vi "Calculator Brainstorming V3.vi"() -> ()   [LabVIEW 2017]
panel:
  in  ".":bool
  in  "÷":bool
  in  "x":bool
  in  "-":bool
  in  "+":bool
  in  "9":bool
  in  "8":bool
  in  "7":bool
  in  "0":bool
  in  "6":bool
  in  "CLEAR":bool
  in  "?":bool
  in  "1":bool
  in  "5":bool
  in  "4":bool
  in  "3":bool
  in  "2":bool
  out "Display":dbl
  # "Don't work:"
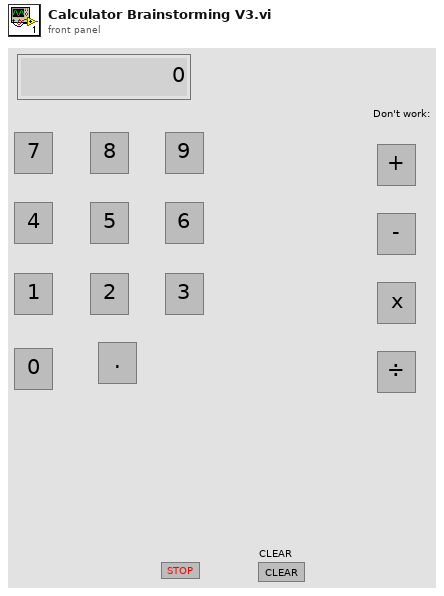
[diagram p1: front panel]
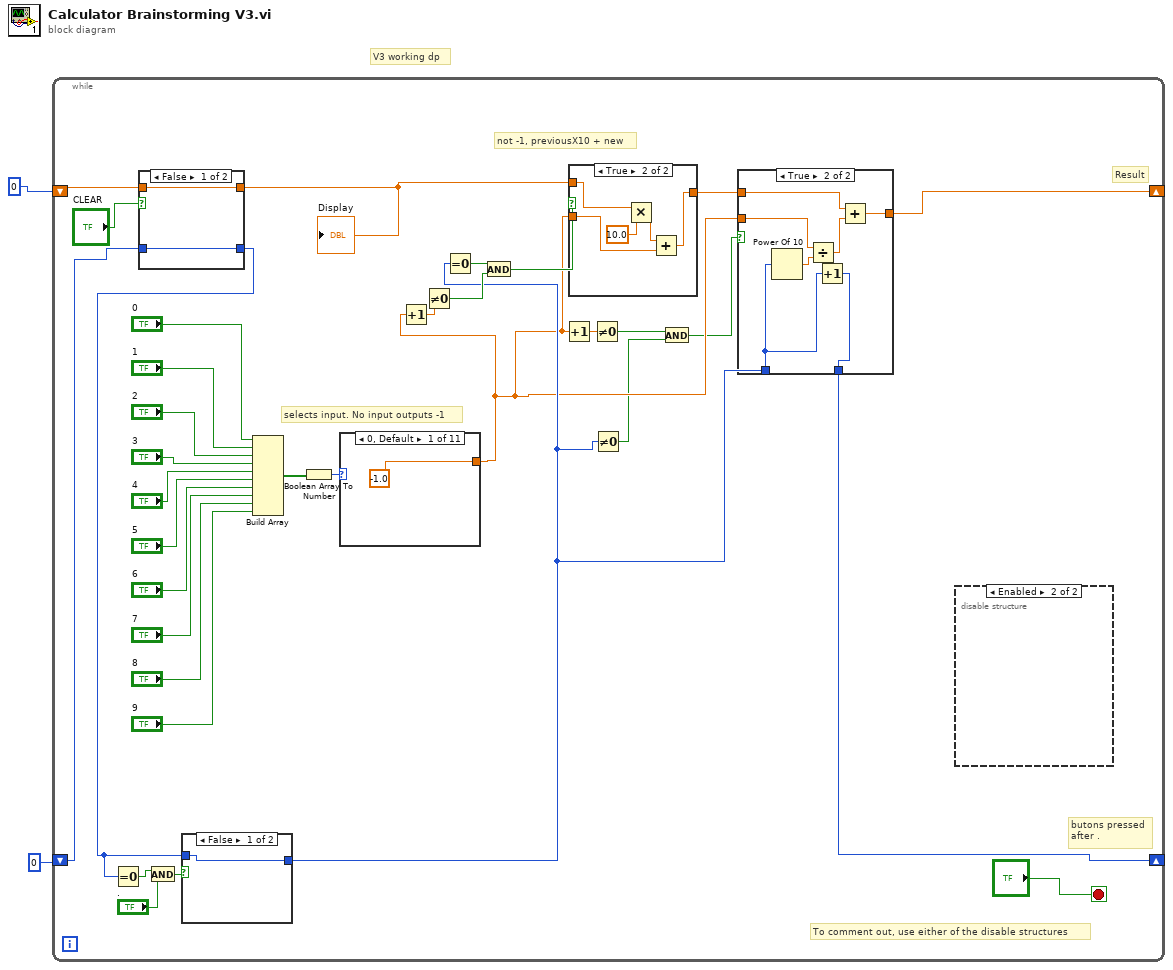
[diagram p0: block diagram]
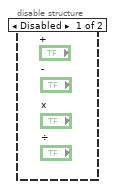
[diagram p2: hidden frame]
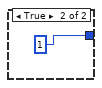
[diagram p5: hidden frame]
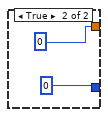
[diagram p6: hidden frame]
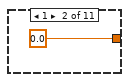
[diagram p7: hidden frame]
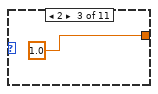
[diagram p8: hidden frame]
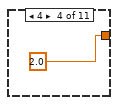
[diagram p9: hidden frame]
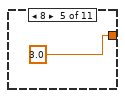
[diagram p10: hidden frame]
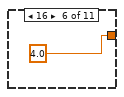
[diagram p11: hidden frame]
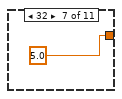
[diagram p12: hidden frame]
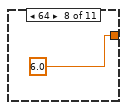
[diagram p13: hidden frame]
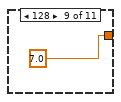
[diagram p14: hidden frame]
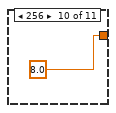
[diagram p15: hidden frame]
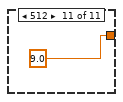
[diagram p16: hidden frame]
diagram:
  # "V3 working dp"
  n1 = while {
    shift-right: [w14] -> _
    shift-left: u8 0 -> [w34]
    shift-right: [w13] -> _
    shift-left: u8 0 -> [w17]
    stop <- "?" stop-if-true
    # "butons pressed\nafter ."
    # "To comment out, use either of the disable structures"
    # "not -1, previousX10 + new"
    # "selects input. No input outputs -1"
    # "Result"
    n2 = case shown="False" "CLEAR" {
      tunnel: [w55 0] -> w16
      tunnel: w34 -> [w55 _]
      tunnel: [w54 0] -> w18
      tunnel: w17 -> [w54 _]
      frame False {
      }
      frame True {
      }
    }
    "Display" <- w16
    n3 = Equal To 0?(x=w18) -> (x = 0?=w20:bool)
    n4 = And(x=w20, y=".") -> (x .and. y?=w21:bool)
    n5 = case shown="False" w21 {
      tunnel: w18 -> [w52 _]
      tunnel: [w52 1] -> w8
      frame False {
      }
      frame True {
      }
    }
    n6 = Build Array("0", "1", "2", "3", "4", "5", "6", "7", "8", "9") -> (w32:bool[])
    n7 = Boolean Array To Number(Boolean array=w32) -> (number=w36:u32)
    n8 = case shown="0, Default" w36 {
      tunnel: [-1.0 0.0 1.0 2.0 3.0 4.0 5.0 6.0 7.0 8.0 9.0] -> w7
      frame 0, Default {
      }
      frame 1 {
      }
      frame 2 {
      }
      frame 4 {
      }
      frame 8 {
      }
      frame 16 {
      }
      frame 32 {
      }
      frame 64 {
      }
      frame 128 {
      }
      frame 256 {
      }
      frame 512 {
      }
    }
    n9 = Increment(x=w7) -> (x+1=w11:dbl)
    n10 = Not Equal To 0?(x=w11) -> (x != 0?=w12:bool)
    n11 = Equal To 0?(x=w8) -> (x = 0?=w10:bool)
    n12 = And(x=w10, y=w12) -> (x .and. y?=w9:bool)
    n13 = Increment(x=w7) -> (x+1=w3:dbl)
    n14 = case shown="True" w9 {
      tunnel: w16 -> [w37 w40]
      tunnel: [w37 w39] -> w15
      tunnel: w7 -> [_ w38]
      frame False {
      }
      frame True {
        n15 = Multiply(x=w40, y=10.0) -> (x*y=w42:dbl)
        n16 = Add(x=w42, y=w38) -> (x+y=w39:dbl)
      }
    }
    n17 = Not Equal To 0?(x=w3) -> (x != 0?=w6:bool)
    n18 = Not Equal To 0?(x=w8) -> (x != 0?=w5:bool)
    n19 = And(x=w6, y=w5) -> (x .and. y?=w4:bool)
    n20 = case shown="True" w4 {
      tunnel: w15 -> [w44 w49]
      tunnel: [w44 w48] -> w14
      tunnel: w8 -> [w43 w46]
      tunnel: w7 -> [_ w47]
      tunnel: [w43 w45] -> w13
      frame False {
      }
      frame True {
        n21 = Power Of 10(x=w46) -> (10^x=w51:dbl)
        n22 = Divide(x=w47, y=w51) -> (x/y=w50:dbl)
        n23 = Increment(x=w46) -> (x+1=w45:i32)
        n24 = Add(x=w49, y=w50) -> (x+y=w48:dbl)
      }
    }
    n25 = disable-structure shown="Enabled" {
      frame Disabled {
      }
      frame Enabled {
      }
    }
  }
